vi "Example.vi"() -> ()   [LabVIEW 2018]
uses:
  <vilib>/DAQmx/create/channels.llb/DAQmx Create Channel (AI-Voltage-Basic).vi
  <vilib>/DAQmx/configure/timing.llb/DAQmx Timing (Sample Clock).vi
  DAQmx Read sim (Analog 1D Wfm NChan NSamp).vi
  DAQmx sim.lvlib
panel:
  out "signals":waveform(dbl)[](graph)
  in  "stop":bool
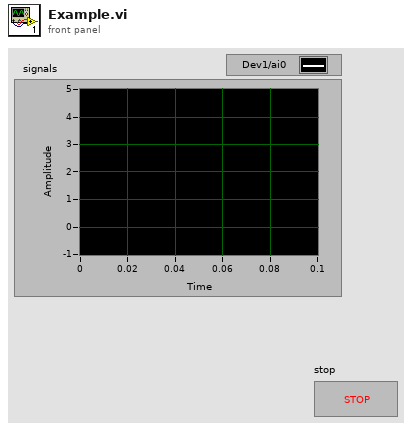
[diagram p1: front panel]
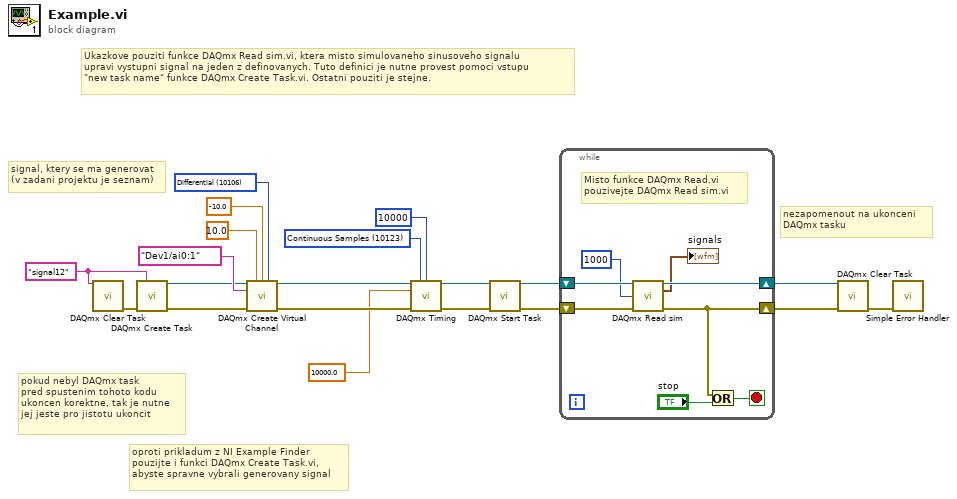
[diagram p0: block diagram]
diagram:
  w1 = "signal12"
  w7 = 10123 items=["Finite Samples"=10178, "Continuous Samples"=10123, "Hardware Timed Single Point"=12522] ("sample mode")
  w8 = 10106 items=["Default"=-1, "RSE"=10083, "NRSE"=10078, "Differential"=10106, "Pseudodifferential"=12529] ("input terminal configuration")
  # "nezapomenout na ukonceni\nDAQmx tasku"
  # "Ukazkove pouziti funkce DAQmx Read sim.vi, ktera misto simulovaneho sinusoveho signalu\nupravi vystupni signal na jeden z definovanych. Tuto definici je nutne provest pomoci vstupu\n\"new task name\" funkce DAQmx Create Task.vi. Ostatni pouziti je stejne."
  # "pokud nebyl DAQmx task\npred spustenim tohoto kodu\nukoncen korektne, tak je nutne\njej jeste pro jistotu ukoncit"
  # "signal, ktery se ma generovat\n(v zadani projektu je seznam)"
  # "oproti prikladum z NI Example Finder\npouzijte i funkci DAQmx Create Task.vi,\nabyste spravne vybrali generovany signal"
  n1 = call <vilib>:"DAQmx Clear Task.vi"("task in"=w1) -> ("error out"=w2:errorcluster)  [unwired: 14 in]
  n2 = call <vilib>:"DAQmx Create Task.vi"("new task name"=w1, "error in"=w2) -> ("task out"=w4:refnum<k21>, "error out"=w3:errorcluster)  [unwired: 12 in]
  n3 = call-poly <vilib>:"DAQmx Create Virtual Channel.vi"("task in"=w4, "maximum value"=10.0, "minimum value"=-10.0, "input terminal configuration"=w8, "physical channels"=tag "Dev1/ai0:1", "error in"=w3) -> ("task out"=w20:refnum<k21>, "error out"=w19:errorcluster)  [unwired: 8 in]
  n4 = call-poly <vilib>:"DAQmx Timing.vi"("task/channels in"=w20, "sample mode"=w7, "samples per channel"=10000, "rate"=10000.0, "error in"=w19) -> ("task out"=w18:refnum<k21>, "error out"=w17:errorcluster)  [unwired: 9 in]
  n5 = call <vilib>:"DAQmx Start Task.vi"("task/channels in"=w18, "error in"=w17) -> ("task out"=w16:refnum<k21>, "error out"=w15:errorcluster)  [unwired: 12 in]
  n6 = while {
    shift-right: [w26] -> w13
    shift-left: w16 -> [w28]
    shift-right: [w22] -> w12
    shift-left: w15 -> [w27]
    stop <- w23 stop-if-true
    # "Misto funkce DAQmx Read.vi\npouzivejte DAQmx Read sim.vi"
    n7 = call-poly "DAQmx Read sim.vi"("task/channels in"=w28, "number of samples per channel"=1000, "error in"=w27) -> ("task out"=w26:refnum<k21>, "data"=→"signals":waveform(dbl)[], "error out"=w22:errorcluster)  [unwired: 10 in]
    n8 = Or(x=w22, y="stop") -> (x .or. y?=w23:bool)
  }
  n9 = call <vilib>:"DAQmx Clear Task.vi"("task in"=w13, "error in"=w12) -> ("error out"=w11:errorcluster)  [unwired: 13 in]
  n10 = call <vilib>:"Simple Error Handler.vi"("error in (no error)"=w11) -> ()  [unwired: 4 in, 5 out]
